vi "RSZVB Set ALC Port Coupling.vi"(8 "error in (no error)":errorcluster {"code" format="%.0x"}, 9 "State (On)":bool=TRUE, 10 "Channel (1)":i32=1, 11 "VISA session":refnum<visa-resource-name>) -> (0 "error out":errorcluster {"code" format="%.0x"}, 3 "dup VISA session":refnum<visa-resource-name>)   [LabVIEW 2011]
doc: "Enforces identical ALC settings for the individual ports in channel <Ch> \n\nRemote-control command(s):\nSOURce<Ch>:POWer:ALC:COUPle"
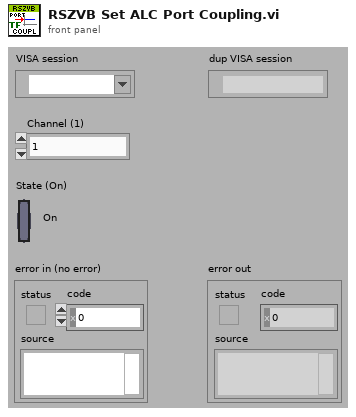
[diagram p1: front panel]
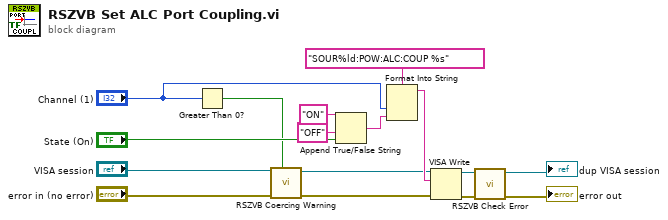
[diagram p0: block diagram]
diagram:
  n1 = Greater Than 0?(x="Channel (1)") -> (x > 0?=w4:bool)
  n2 = call "RSZVB Coercing Warning.vi"("In Range?"=w4, "error in (no error)"="error in (no error)", "VISA session"="VISA session") -> ("error out"=w9:errorcluster, "dup VISA session"=w10:refnum<visa-resource-name>)  [unwired: 7 in]
  n3 = Append True/False String(1:"State (On)", 2:"OFF" ("false string"), 3:"ON" ("true string")) -> (0:w1:string)  [unwired: 1 in]
  n4 = Format Into String(format string="SOUR%ld:POW:ALC:COUP %s", "Channel (1)", w1) -> (resulting string=w13:string)  [unwired: 2 in, 1 out]
  n5 = VISA Write(VISA resource name=w10, write buffer=w13, error in (no error)=w9) -> (VISA resource name out=w11:refnum<visa-resource-name>, error out=w12:errorcluster)  [unwired: 1 out]
  n6 = call "RSZVB Check Error.vi"("error in (no error)"=w12, "VISA session"=w11) -> ("error out"=→"error out":errorcluster, "dup VISA session"=→"dup VISA session":refnum<visa-resource-name>)  [unwired: 8 in]
